vi "Read System Status.vi"(8 "error in (no error)":errorcluster, 11 "System in":refnum<class "System.lvclass">) -> (0 "error out":errorcluster, 2 "System Status":T1, 3 "System out":refnum<class "System.lvclass">)   [LabVIEW 2013, in "System.lvlib" / "System.lvclass"]
uses:
  System.lvclass
  System Status.ctl
  SystemStates.ctl
  Command Processor/Command Processor Status.ctl
  Current Previous State Status.ctl
  State Status.ctl
  Command Processor/Command/Command Status.ctl
  Command Processor/Command/State Status.ctl
  System.lvclass/System.ctl
  Command Processor/Command Processor.lvclass
  Command Processor/Command/Command.lvclass
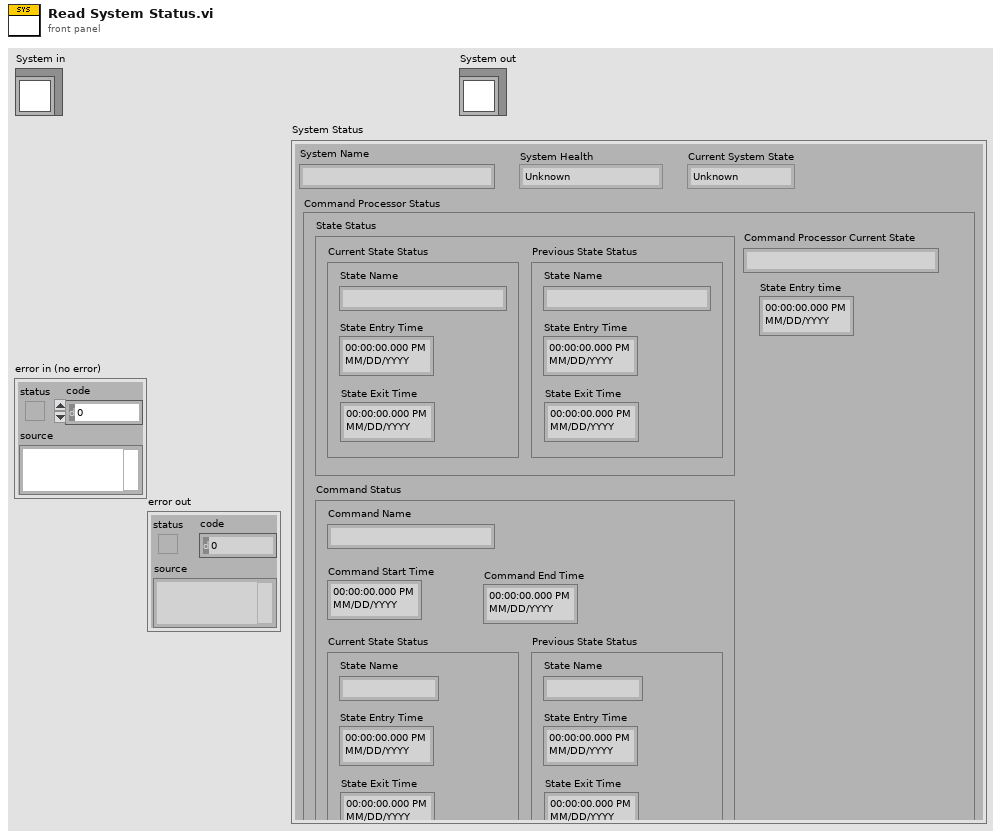
[diagram p1: front panel]
types:
  T1 = typedef "System.lvlib/System.lvclass/System Status.ctl" = cluster{"Current System State":T2, "System Health":enum16{"Unknown", "Good", "Poor", "Bad"}, "System Name":string, "Command Processor Status":T3}
  T2 = typedef "System.lvlib/System.lvclass/SystemStates.ctl" = enum16{"Unknown", "Running", "Stopped"}
  T3 = typedef "Command Processor.lvlib/Command Processor.lvclass/Command Processor Status.ctl" = cluster{"State Entry time":timestamp, "State Status":T4, "Command Processor Current State":string, "Command Status":T6}
  T4 = typedef "Current Previous State Status.ctl" = cluster{"Current State Status":T5, "Previous State Status":T5}
  T5 = typedef "State Status.ctl" = cluster{"State Name":string, "State Entry Time":timestamp, "State Exit Time":timestamp}
  T6 = typedef "Command Processor.lvlib/Command.lvlib/Command.lvclass/Command Status.ctl" = cluster{"Command Name":string, "Current State Status":T7, "Command Start Time":timestamp, "Command End Time":timestamp, "Previous State Status":T7}
  T7 = typedef "Command Processor.lvlib/Command.lvlib/Command.lvclass/State Status.ctl" = cluster{"State Name":string, "State Entry Time":timestamp, "State Exit Time":timestamp}
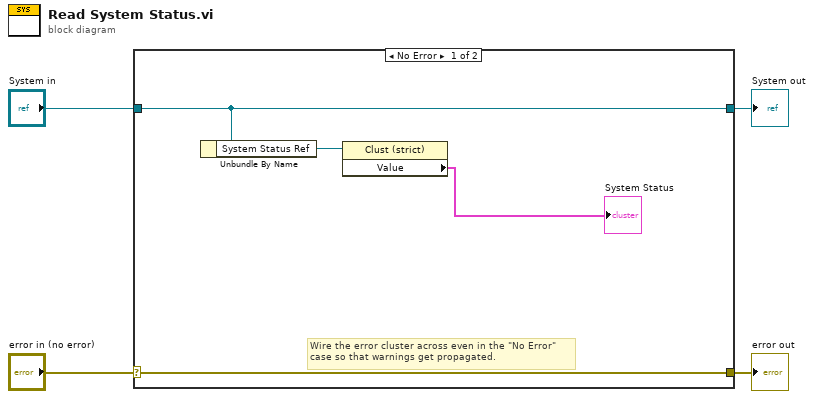
[diagram p0: block diagram]
diagram:
  n1 = case shown="No Error" "error in (no error)" {
    selector: "error in (no error)" -> [w8 w10]
    tunnel: [w8 w10] -> w3
    tunnel: [w7 w9] -> w1
    tunnel: "System in" -> [w7 w9]
    frame No Error {
      # "Wire the error cluster across even in the \"No Error\"\ncase so that warnings get propagated."
      n2 = Unbundle By Name(w7) -> ("System Status Ref"=w6:refnum<vi>)
      n3 = property class="Clust (strict)"(reference=w6) -> ("Value"=→"System Status":T1)  [unwired: 1 in, 2 out]
    }
    frame Error {
    }
  }
  "error out" <- w3
  "System out" <- w1
